vi "PCO_GetNoiseFilterMode.vi"(8 "error in (no error)":errorcluster {"code" format="%x"}, 11 "ph":u64) -> (0 "error out":errorcluster {"code" format="%x"}, 1 "wNoiseFilterMode":u16(ring) items=["OFF", "ON"], 2 "ErrorMessage":i32 format="%x", 3 "ph out":u64)   [LabVIEW 2019, in "SDK.lvlib" / "ImageSensor.lvlib"]
doc: "<b>Description:</b>\nThis function returns the current operating mode of the image correction in the camera.\n\n<b>Supported camera type:</b>\nAll cameras\n\n<b>Descriptor dependency:</b>\ndwGeneralCapsDESC1: NOISE_FILTER, HOTPIX_ONLY_WITH_NOISE_FILTER"
uses:
  ImageSensor.lvlib
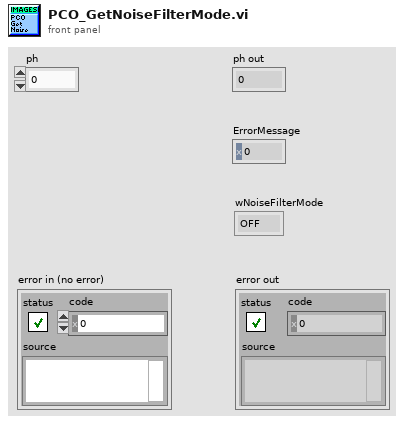
[diagram p1: front panel]
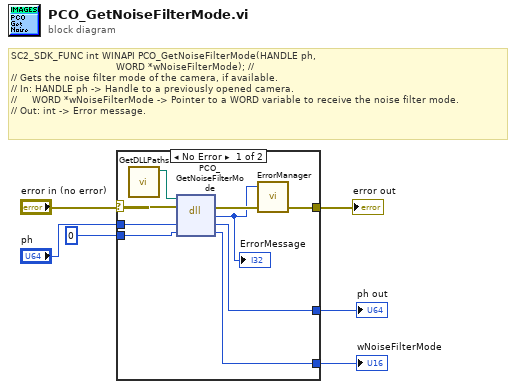
[diagram p0: block diagram]
diagram:
  # "SC2_SDK_FUNC int WINAPI PCO_GetNoiseFilterMode(HANDLE ph,\n                                   WORD *wNoiseFilterMode); // \n// Gets the noise filter mode of the camera, if available.\n// In: HANDLE ph -> Handle to a previously opened camera.\n//     WORD *wNoiseFilterMode -> Pointer to a WORD variable to receive the noise filter mode.\n// Out: int -> Error message."
  n1 = case shown="No Error" "error in (no error)" {
    selector: "error in (no error)" -> [w8 w18]
    tunnel: "ph" -> [w15 w17]
    tunnel: [w14 w17] -> w5
    tunnel: u16 0 ("wNoiseFilterMode") -> [w13 w16]
    tunnel: [w12 w16] -> w3
    tunnel: [w10 w18] -> w2
    frame No Error {
      n2 = call "GetDLLPaths.vi"() -> ("SC2_Cam_Path"=w7:path)  [unwired: 8 in, 3 out]
      n3 = dll-call lib="?" fn="PCO_GetNoiseFilterMode"(path in=w7, error in=w8, "ph"=w15, "wNoiseFilterMode"=w13) -> (error out=w11:errorcluster, "return type"=w9:i32, "ph"=w14:u64, "wNoiseFilterMode"=w12:u16)  [unwired: 1 in, 1 out]
      "ErrorMessage" <- w9
      n4 = call "ErrorManager.vi"("error in (no error)"=w11, "error code"=w9) -> ("error out"=w10:errorcluster)  [unwired: 2 in, 1 out]
    }
    frame Error {
    }
  }
  "ph out" <- w5
  "wNoiseFilterMode" <- w3
  "error out" <- w2
